vi "GVSDataView Mark Frame Right.vi"() -> ()   [LabVIEW 2013]
uses:
  <vilib>/Utility/miscctls.llb/LVPositionTypeDef.ctl
  SubVI/GVSMain Sub Window Global.vi
  GVSNew View Global.vi
panel:
  in  "sMe":string
  in  "bShow":bool=TRUE
  in  "Right":bool
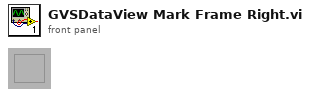
[diagram p1: front panel]
types:
  T1 = typedef "LVPositionTypeDef.ctl" = cluster{"Left":i32, "Top":i32}
  T2 = typedef "LVRectTypeDef.ctl" = cluster{"Left":i16, "Top":i16, "Right":i16, "Bottom":i16}
  T3 = typedef "Graph Main Info Cluster.ctl" = cluster{"Selected_BarIdx":i32, "Selected_PanelIdx":i32, "Graph Main VIRef":refnum<vi>, "ToolBarClick":bool, "Spliter Ref Array":refnum<vi>[], "Panel Ref Array":refnum<vi>[], "Spliter_matrix":i32[][], "Panel_matrix":i32[][], "child_spliterIdx_matrix":i32[][], "split_pos_matrix":i32[][], "Title State":bool, "sQueueName":string, "Frame nID":i32, "Graph VIRef Array":cluster{"Graph VIRef":refnum<vi>, "Panel Idx":i32, "Frame VIRef":refnum<vi>, "Icon Ring":i32, "Graph Type":string}[], "View Type":string}
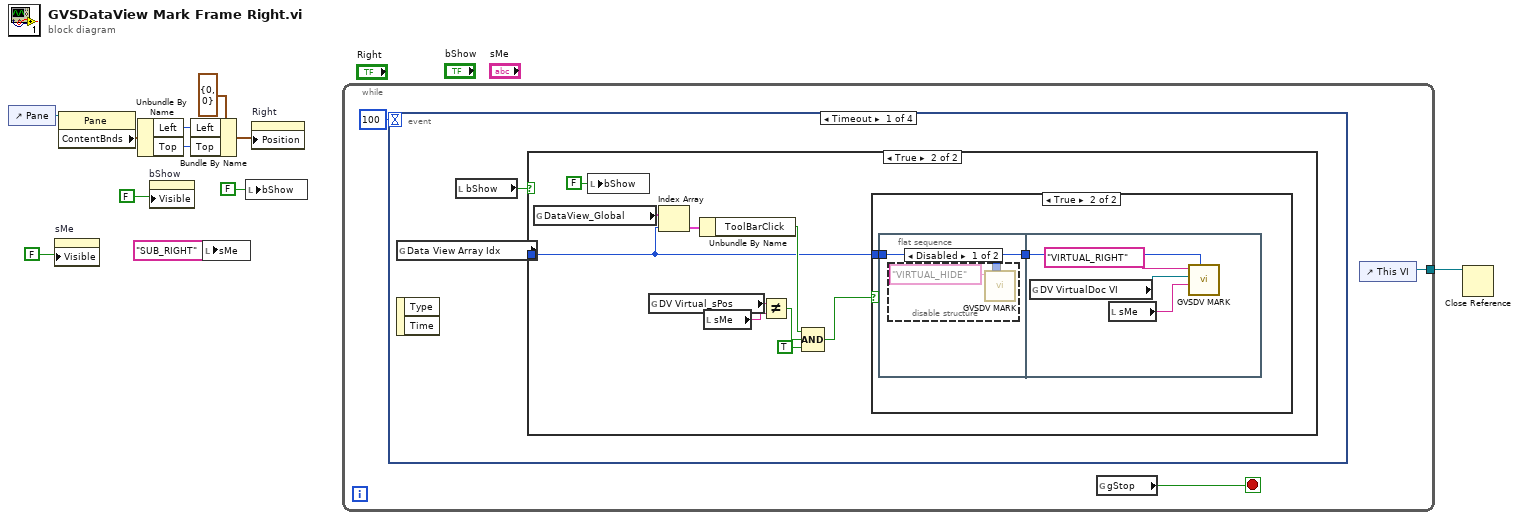
[diagram p0: block diagram]
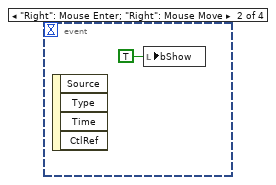
[diagram p5: hidden frame]
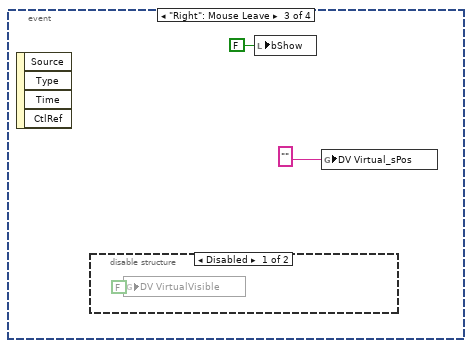
[diagram p6: hidden frame]
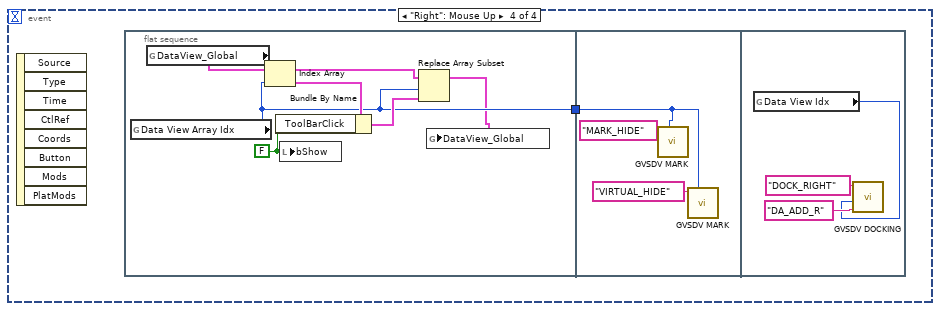
[diagram p8: hidden frame]
diagram:
  n1 = control-ref of="Pane"() -> (w11:refnum<vi>)
  n2 = property on="sMe" class="Str"("Visible"=FALSE) -> ()  [unwired: 2 in, 2 out]
  n3 = property class="Pane"(reference=w11) -> ("ContentBnds"=w10:T2)  [unwired: 1 in, 2 out]
  n4 = Unbundle By Name(w10) -> ("Left"=w9:i16, "Top"=w7:i16)
  n5 = property on="bShow" class="Bool (strict)"("Visible"=FALSE) -> ()  [unwired: 2 in, 2 out]
  n6 = Bundle By Name(cluster=T1 {"Left"=0, "Top"=0} ("Position"), "Left"=w9, "Top"=w7) -> (w6:T1)
  n7 = local write "sMe"("SUB_RIGHT" ("sMe")) -> ()
  n8 = local write "bShow"(FALSE ("bShow")) -> ()
  n9 = property on="Right" class="Bool (strict)"("Position"=w6) -> ()  [unwired: 2 in, 2 out]
  n10 = while {
    tunnel: [w13] -> w1
    stop <- w12 stop-if-true
    n11 = event shown="[0] Timeout" {
      selector: _ -> [_ _ _ _]
      dyn-events: _ -> [_ _ _ _]
      timeout: 100 -> [_ _ _ _]
      event Timeout {
        n12 = global read "GVSNew View Global.vi" "Data View Array Idx"() -> (w15:i32)
        n13 = event-data() -> ()  [unwired: 3 out]
        n14 = local read "bShow"() -> (w16:bool)
        n15 = case shown="True" w16 {
          tunnel: w15 -> [_ w18]
          frame False {
          }
          frame True {
            n16 = global read "GVSNew View Global.vi" "DataView_Global"() -> (w22:T3[])
            n17 = local write "bShow"(FALSE ("bShow")) -> ()
            n18 = global read "GVSNew View Global.vi" "DV Virtual_sPos"() -> (w26:string)
            n19 = Index Array(array=w22, index=w18) -> (element=w23:T3)
            n20 = Unbundle By Name(w23) -> ("ToolBarClick"=w21:bool)
            n21 = local read "sMe"() -> (w25:string)
            n22 = Not Equal?(x=w26, y=w25) -> (x != y?=w20:bool)
            n23 = Compound Arithmetic op=AND(w21, w20, TRUE ("value")) -> (w24:bool)
            n24 = case shown="True" w24 {
              tunnel: w18 -> [_ w28]
              frame False {
              }
              frame True {
                n25 = flat-sequence {
                  tunnel: w28 -> [w29]
                  tunnel: [w29] -> w27
                  tunnel: w27 -> [w32]
                  frame #0 {
                    n26 = disable-structure shown="Disabled" {
                      disable-tunnel: w29 -> [w31 _]
                      frame Disabled {
                        n27 = call "GVSDV MARK.vi"("sAction"="VIRTUAL_HIDE", "DataView Array Index"=w31) -> ()  [unwired: 8 in, 1 out]
                      }
                      frame Enabled {
                      }
                    }
                  }
                  frame #1 {
                    n28 = global read "GVSNew View Global.vi" "DV VirtualDoc VI"() -> (w33:refnum<vi>)
                    n29 = local read "sMe"() -> (w34:string)
                    n30 = call "GVSDV MARK.vi"("sAction"="VIRTUAL_RIGHT", "mVritual_VIRef"=w33, "sData"=w34, "DataView Array Index"=w32) -> ()  [unwired: 6 in, 1 out]
                  }
                }
              }
            }
          }
        }
      }
      event "Right": Mouse Enter; "Right": Mouse Move {
        n31 = event-data() -> ()  [unwired: 5 out]
        n32 = local write "bShow"(TRUE ("bShow")) -> ()
      }
      event "Right": Mouse Leave {
        n33 = event-data() -> ()  [unwired: 5 out]
        n34 = disable-structure shown="Disabled" {
          frame Disabled {
            n35 = global write "GVSNew View Global.vi" "DV VirtualVisible"(FALSE ("VirtualVi")) -> ()
          }
          frame Enabled {
          }
        }
        n36 = local write "bShow"(FALSE ("bShow")) -> ()
        n37 = global write "GVSNew View Global.vi" "DV Virtual_sPos"("" ("Virtual_sPos")) -> ()
      }
      event "Right": Mouse Up {
        n38 = event-data() -> ()  [unwired: 9 out]
        n39 = flat-sequence {
          tunnel: [w42] -> w40
          tunnel: w40 -> [w48]
          frame #0 {
            w45 = FALSE ("bShow")
            n40 = global read "GVSNew View Global.vi" "Data View Array Idx"() -> (w42:i32)
            n41 = global read "GVSNew View Global.vi" "DataView_Global"() -> (w43:T3[])
            n42 = Index Array(array=w43, index=w42) -> (element=w46:T3)
            n43 = Bundle By Name(cluster=w46, "ToolBarClick"=w45) -> (w44:T3)
            n44 = local write "bShow"(w45) -> ()
            n45 = Replace Array Subset(array=w43, new element=w44, index=w42) -> (w41:T3[])
            n46 = global write "GVSNew View Global.vi" "DataView_Global"(w41) -> ()
          }
          frame #1 {
            n47 = call "GVSDV MARK.vi"("sAction"="MARK_HIDE", "DataView Array Index"=w48) -> ()  [unwired: 8 in, 1 out]
            n48 = call "GVSDV MARK.vi"("sAction"="VIRTUAL_HIDE", "DataView Array Index"=w48) -> ()  [unwired: 8 in, 1 out]
          }
          frame #2 {
            n49 = global read "GVSNew View Global.vi" "Data View Idx"() -> (w50:i32)
            n50 = call "GVSDV DOCKING.vi"("sData"="DA_ADD_R" ("Action Type"), "DataView Index"=w50, "sAction"="DOCK_RIGHT") -> ()  [unwired: 5 in, 4 out]
          }
        }
      }
    }
    n51 = global read "GVSMain Sub Window Global.vi" "gStop"() -> (w12:bool)
    n52 = control-ref of="This VI"() -> (w13:refnum<vi>)
  }
  n53 = Close Reference(reference=w1) -> ()  [unwired: 1 in, 1 out]
